vi "WPI_DashboardPublish Commands.vi"(8 "error in (no error)":errorcluster) -> (0 "error out":errorcluster)   [LabVIEW 2017]
doc: "Walk through VIs discovering who has Command Info on their connector and seems to be a test.\nAdd them to the list of Commands that will show on the Commands tab."
uses:
  <vilib>/Utility/Data Type/NI_Data Type.lvlib
panel:
  out "x-y":u32
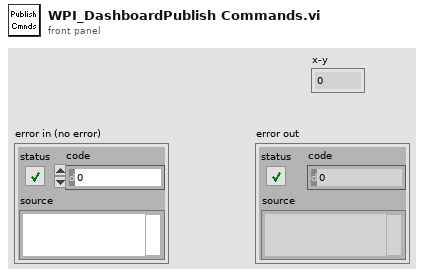
[diagram p1: front panel]
types:
  T1 = typedef "NI_Data Type.lvlib/Type Definition Info.ctl" = cluster{"Name":string, "Timestamp":u32}
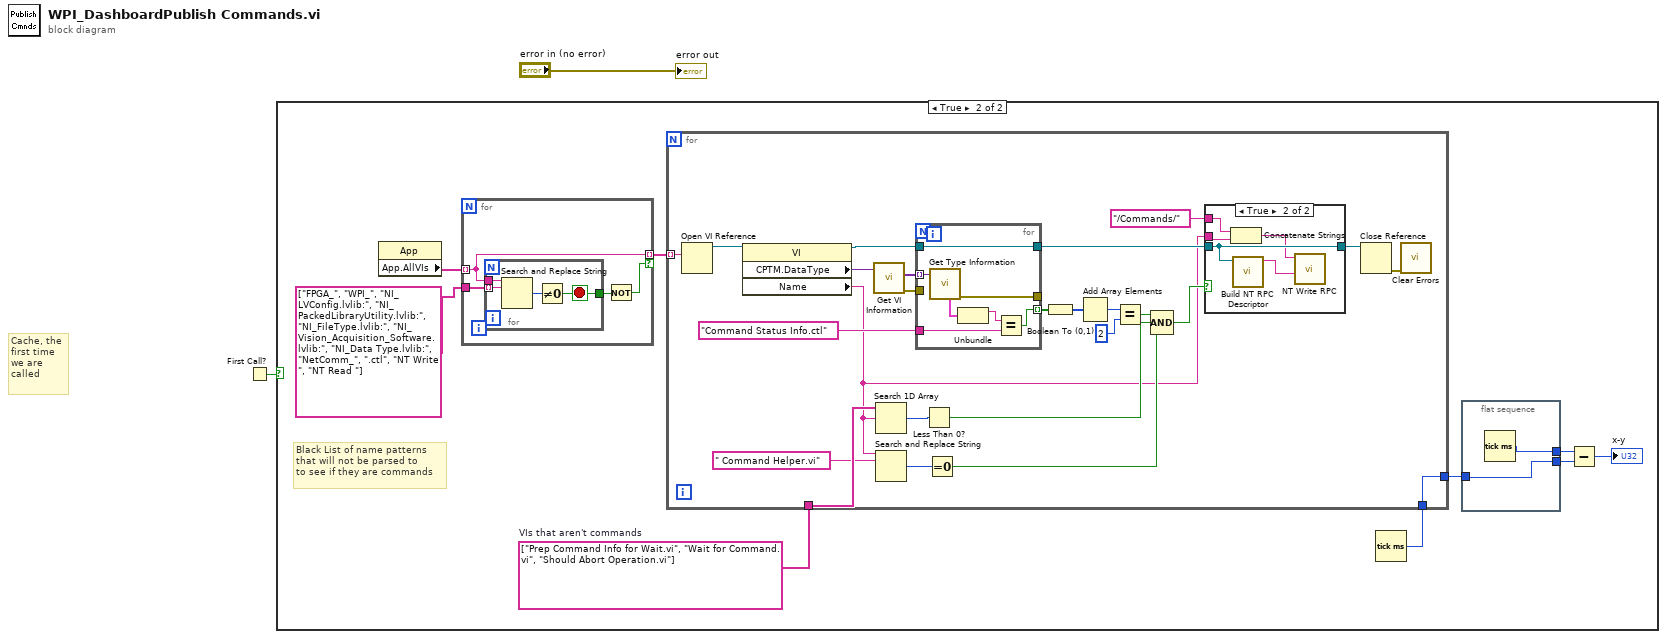
[diagram p0: block diagram]
diagram:
  # "Cache, the\nfirst time\nwe are\ncalled"
  n1 = First Call?() -> (First Call?: T/F=w1:bool)
  n2 = case shown="True" w1 {
    frame False {
    }
    frame True {
      w11 = string[] ["Prep Command Info for Wait.vi", "Wait for Command.vi", "Should Abort Operation.vi"]  # VIs that aren't commands
      # "Black List of name patterns\nthat will not be parsed to\nto see if they are commands"
      n3 = property class="App"() -> ("App.AllVIs"=w5:string[])  [unwired: 2 in, 2 out]
      n4 = for {
        tunnel: w5 -> [w14] mode=indexing
        tunnel: string[] ["FPGA_", "WPI_", "NI_LVConfig.lvlib:", "NI_PackedLibraryUtility.lvlib:", "NI_FileType.lvlib:", "NI_Vision_Acquisition_Software.lvlib:", "NI_Data Type.lvlib:", "NetComm_", ".ctl", "NT Write ", "NT Read "] -> [w15]
        tunnel: [w14] -> w4 mode=indexing if=w12
        n5 = for {
          tunnel: w15 -> [w19] mode=indexing
          tunnel: w14 -> [w18]
          tunnel: [w16] -> w13
          stop <- w16 stop-if-true
          n6 = Search and Replace String(input string=w18, search string=w19) -> (number of replacements=w17:i32)  [unwired: 6 in, 3 out]
          n7 = Not Equal To 0?(x=w17) -> (x != 0?=w16:bool)
        }
        n8 = Not(x=w13) -> (.not. x?=w12:bool)
      }
      n9 = Tick Count (ms)() -> (millisecond timer value=w10:u32)
      n10 = for {
        tunnel: w4 -> [w46] mode=indexing
        tunnel: w11 -> [w45]
        tunnel: w10 -> [w44]
        tunnel: [w44] -> w9
        n11 = Open VI Reference(vi path=w46) -> (vi reference=w25:refnum<vi>)  [unwired: 5 in, 1 out]
        n12 = property class="VI"(reference=w25) -> (reference out=w24:refnum<vi>, "CPTM.DataType"=w22:variant, "Name"=w23:string)  [unwired: 1 in, 1 out]
        n13 = call <vilib>:"Get VI Information.vi"("Variant"=w22) -> ("error out"=w29:errorcluster, "VI Terminal Types"=w30:variant[])  [unwired: 7 in, 2 out]
        n14 = Search 1D Array(1D array=w45, element=w23) -> (index of element=w42:i32)  [unwired: 1 in]
        n15 = Search and Replace String(input string=w23, search string=" Command Helper.vi") -> (number of replacements=w39:i32)  [unwired: 6 in, 3 out]
        n16 = for {
          tunnel: "Command Status Info.ctl" ("Name") -> [w59]
          tunnel: [w58] -> w35 mode=indexing
          tunnel: [w57] -> w27
          tunnel: w24 -> [w57]
          tunnel: w30 -> [w56] mode=indexing
          tunnel: w29 -> [_]
          tunnel: [w55] -> _
          n17 = call <vilib>:"Get Type Information.vi"("Variant"=w56) -> ("error out"=w55:errorcluster, "Type Definition Info"=w54:T1)  [unwired: 6 in, 3 out]
          n18 = Unbundle(w54) -> ("Name"=w53:string)  [unwired: 1 out]
          n19 = Equal?(x=w53, y=w59) -> (x = y?=w58:bool)
        }
        n20 = Less Than 0?(x=w42) -> (x < 0?=w41:bool)
        n21 = Equal To 0?(x=w39) -> (x = 0?=w38:bool)
        n22 = Boolean To (0,1)(Boolean=w35) -> (0, 1=w34:i16[])
        n23 = Add Array Elements(numeric array=w34) -> (sum=w33:i16)
        n24 = Equal?(x=w33, y=2) -> (x = y?=w31:bool)
        n25 = Compound Arithmetic op=AND(w31, w41, w38) -> (w28:bool)
        n26 = case shown="True" w28 {
          tunnel: w27 -> [w47 w52]
          tunnel: [w47 w52] -> w36
          tunnel: w23 -> [_ w48]
          tunnel: "/Commands/" -> [_ w50]
          frame False {
          }
          frame True {
            n27 = Concatenate Strings(w50, w48) -> (w49:string)
            n28 = call <vilib>:"Build NT RPC Descriptor.vi"("VI in"=w52) -> ("string buffer"=w51:string)  [unwired: 10 in]
            n29 = call <vilib>:"NT Write RPC.vi"("Buffer"=w51, "Name"=w49) -> ()  [unwired: 9 in, 1 out]
          }
        }
        n30 = Close Reference(reference=w36) -> (error out=w37:errorcluster)  [unwired: 1 in]
        n31 = call <vilib>:"Clear Errors.vi"("error in (no error)"=w37) -> ()  [unwired: 5 in, 2 out]
      }
      n32 = flat-sequence {
        tunnel: w9 -> [w20]
        tunnel: [w21] -> w8
        tunnel: [w20] -> w7
        frame #0 {
          n33 = Tick Count (ms)() -> (millisecond timer value=w21:u32)
        }
      }
      n34 = Subtract(x=w8, y=w7) -> (x-y=→"x-y":u32)
    }
  }
  "error out" <- "error in (no error)"
